vi "Get Status.vi"(8 "error in (no error)":errorcluster, 11 "Actor API in":refnum<class "Actor API.lvclass">) -> (0 "error out":errorcluster, 3 "Status":string)   [LabVIEW 2020, in "RTAF.lvlib" / "Actor API.lvclass"]
uses:
  Actor API.lvclass
  RTAF.lvlib
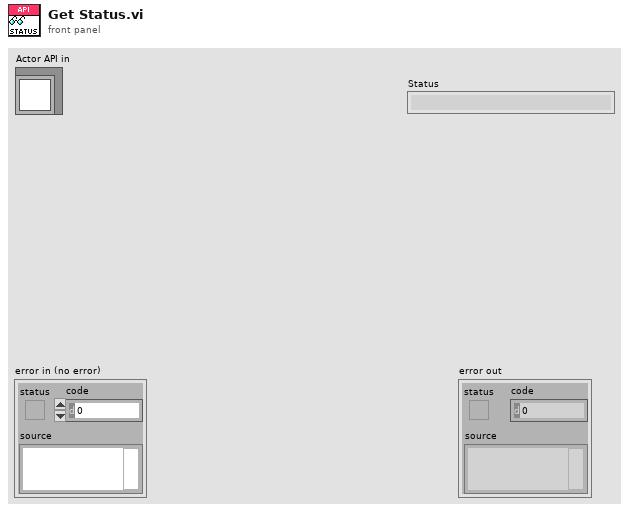
[diagram p1: front panel]
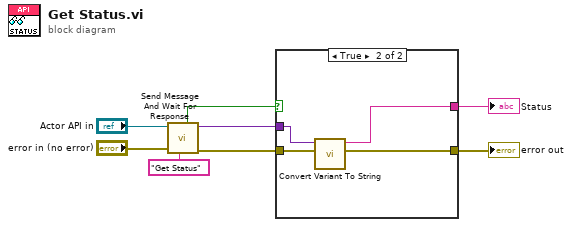
[diagram p0: block diagram]
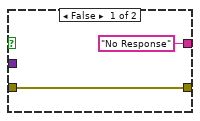
[diagram p2: hidden frame]
diagram:
  n1 = call "Send Message And Wait For Response.vi"("Name"="Get Status", "error in (no error)"="error in (no error)", "Actor API in"="Actor API in") -> ("error out"=w5:errorcluster, "Response"=w3:variant, "Response Received"=w4:bool)  [unwired: 6 in]
  n2 = case shown="True" w4 {
    tunnel: w5 -> [w10 w14]
    tunnel: w3 -> [_ w13]
    tunnel: [w10 w12] -> w2
    tunnel: ["No Response" ("String") w11] -> w1
    frame False {
    }
    frame True {
      n3 = call "Convert Variant To String.vi"("error in (no error)"=w14, "Variant"=w13) -> ("error out"=w12:errorcluster, "String"=w11:string)  [unwired: 8 in]
    }
  }
  "error out" <- w2
  "Status" <- w1
